vi "BLINKING LED USING DAQ.vi"() -> ()   [LabVIEW 2018]
panel:
  in  "stop":bool
  in  "Boolean 3":bool
  in  "Boolean 2":bool
  in  "Boolean":bool
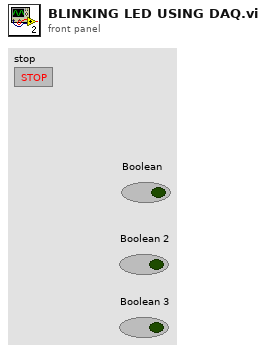
[diagram p1: front panel]
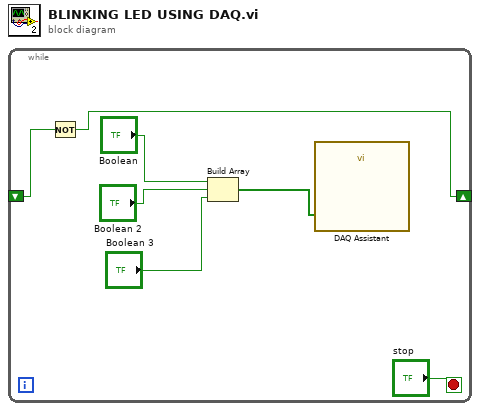
[diagram p0: block diagram]
diagram:
  n1 = while {
    shift-right: [w3] -> _
    shift-left: _ -> [w2]
    stop <- "stop" stop-if-true
    n2 = Not(x=w2) -> (.not. x?=w3:bool)
    n3 = Build Array("Boolean", "Boolean 2", "Boolean 3") -> (w4:bool[])
    n4 = call "DAQ Assistant"("data"=w4) -> ()  [unwired: 17 in, 2 out]
  }
